vi "merge configuration with system.vi"(8 "error in":errorcluster, 11 "Scan Engine configuration in":refnum<class "Scan Engine configuration.lvclass">) -> (0 "error out":errorcluster, 3 "Scan Engine configuration out":refnum<class "Scan Engine configuration.lvclass">)   [LabVIEW 2014, in "Scan Engine runtime.lvclass"]
uses:
  Scan Engine runtime.lvclass
  <vilib>/NI/Tag Bus Module Framework/channel/channel classification.ctl
  <vilib>/NI/Tag Bus Module Framework/channel/TBM channel.lvclass
  configuration/Line.ctl
  configuration/Scan Engine configuration.lvclass
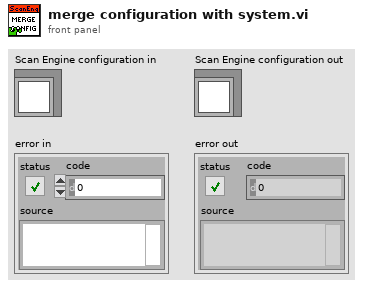
[diagram p1: front panel]
types:
  T1 = typedef "Scan Engine runtime.lvclass/system variable.ctl" = cluster{"reference":refnum<k21>, "data type":T2, "Writable":bool}
  T2 = typedef "tag bus.lvlib/tag descriptor.lvclass/Data Type.ctl" = enum16{"Double", "Single", "I64", "I32", "I16", "I8", "U64", "U32", "U16", "U8", "Boolean", "String", "Array of Double", "Array of Single", "Array of I64", "Array of I32", "Array of I16", "Array of I8", "Array of U64", "Array of U32", "Array of U16", "Array of U8", "Array of Boolean", "Array of String"}
  T3 = typedef "Scan Engine configuration.lvclass/Line.ctl" = cluster{"channel":refnum<class "TBM channel.lvclass">, "Tag":string}
  T4 = typedef "TBM channel.lvclass/channel classification.ctl" = enum16{"input data", "output data", "processing parameter", "processing result"}
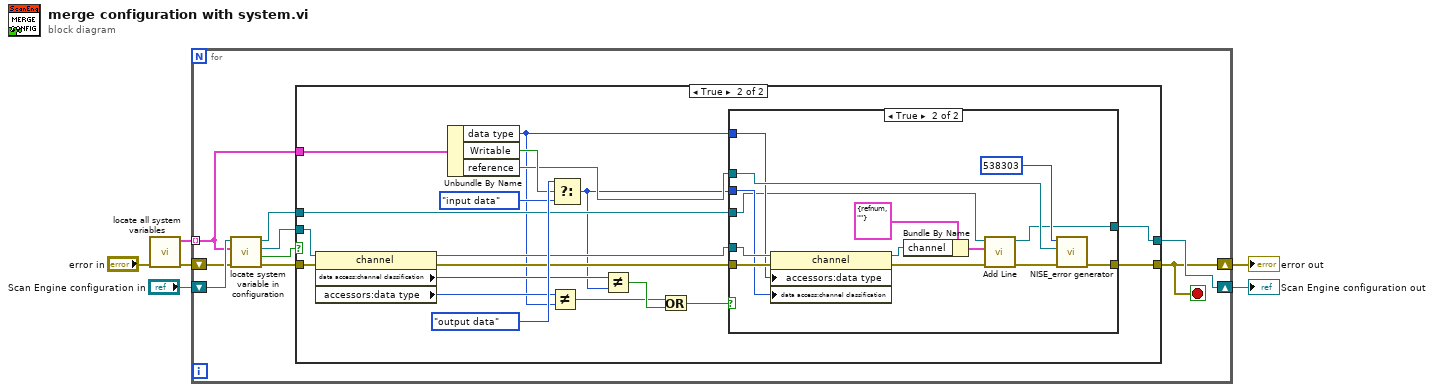
[diagram p0: block diagram]
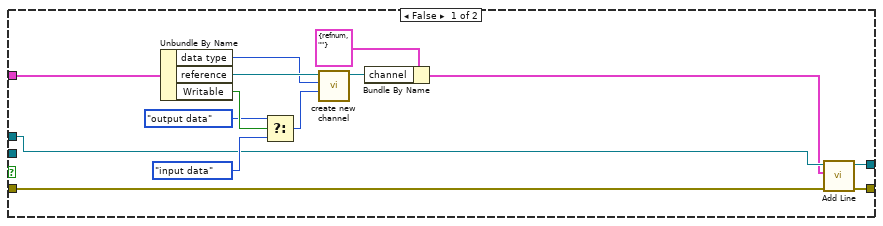
[diagram p2: hidden frame]
diagram:
  n1 = call "locate all system variables.vi"("error in"="error in") -> ("error out"=w1:errorcluster, "system variables"=w3:T1[])  [unwired: 9 in]
  n2 = for {
    shift-right: [w8] -> w5
    shift-left: "Scan Engine configuration in" -> [w15]
    shift-right: [w7] -> w4
    shift-left: w1 -> [w14]
    tunnel: w3 -> [w9] mode=indexing
    stop <- w7 stop-if-true
    n3 = call "locate system variable in configuration.vi"("error in"=w14, "raw variable data"=w9, "Scan Engine configuration in"=w15) -> ("error out"=w12:errorcluster, "found?"=w13:bool, "channel"=w10:refnum<class "TBM channel.lvclass">, "Scan Engine configuration out"=w11:refnum<class "Scan Engine configuration.lvclass">)  [unwired: 5 in]
    n4 = case shown="True" w13 {
      tunnel: w12 -> [w28 w44]
      tunnel: w11 -> [w18 w36]
      tunnel: w10 -> [_ w43]
      tunnel: w9 -> [w29 w48]
      tunnel: [w16 w34] -> w7
      tunnel: [w19 w37] -> w8
      frame False {
        n5 = Unbundle By Name(w29) -> ("data type"=w22:T2, "reference"=w23:refnum<k21>, "Writable"=w27:bool)
        n6 = Select(t=channel_classification."output data" ("channel classification"), s=w27, f=channel_classification."input data" ("channel classification")) -> (s? t:f=w24:T4)
        n7 = call <vilib>:"create new channel.vi"("channel classification"=w24, "data type"=w22, "channel name"=w23) -> ("channel"=w20:refnum<class "TBM channel.lvclass">)  [unwired: 8 in]
        n8 = Bundle By Name(cluster=T3 {"channel"=refnum, "Tag"=""} ("Line"), "channel"=w20) -> (w17:T3)
        n9 = call "Add Line.vi"("error in"=w28, "Line"=w17, "Scan Engine configuration in"=w18) -> ("error out"=w16:errorcluster, "Scan Engine configuration out"=w19:refnum<class "Scan Engine configuration.lvclass">)  [unwired: 7 in]
      }
      frame True {
        n10 = property class="channel"(reference=w43, error in=w44) -> (reference out=w32:refnum<class "TBM channel.lvclass">, error out=w35:errorcluster, "data access:channel classification"=w41:T4, "accessors:data type"=w42:T2)
        n11 = Unbundle By Name(w48) -> ("data type"=w30:T2, "Writable"=w45:bool, "reference"=w33:refnum<k21>)
        n12 = Not Equal?(x=w42, y=w30) -> (x != y?=w39:bool)
        n13 = Select(t=channel_classification."output data" ("channel classification"), s=w45, f=channel_classification."input data" ("channel classification")) -> (s? t:f=w31:T4)
        n14 = Not Equal?(x=w41, y=w31) -> (x != y?=w40:bool)
        n15 = Or(x=w39, y=w40) -> (x .or. y?=w38:bool)
        n16 = case shown="True" w38 {
          tunnel: [w50 w56] -> w37
          tunnel: w36 -> [w50 w57]
          tunnel: w35 -> [w49 w60]
          tunnel: [w49 w63] -> w34
          tunnel: w33 -> [_ w62]
          tunnel: w32 -> [_ w61]
          tunnel: w31 -> [_ w58]
          tunnel: w30 -> [_ w59]
          frame False {
          }
          frame True {
            n17 = property class="channel"(reference=w61, error in=w60, "accessors:data type"=w59, "data access:channel classification"=w58) -> (reference out=w54:refnum<class "TBM channel.lvclass">, error out=w52:errorcluster)
            n18 = Bundle By Name(cluster=T3 {"channel"=refnum, "Tag"=""} ("Line"), "channel"=w54) -> (w53:T3)
            n19 = call "Add Line.vi"("error in"=w52, "Line"=w53, "Scan Engine configuration in"=w57) -> ("error out"=w51:errorcluster, "Scan Engine configuration out"=w56:refnum<class "Scan Engine configuration.lvclass">)  [unwired: 7 in]
            n20 = call <vilib>:"NISE_error generator.vi"("error in"=w51, "append error message"=w62, "error code (0)"=538303) -> ("error out"=w63:errorcluster)  [unwired: 6 in]
          }
        }
      }
    }
  }
  "Scan Engine configuration out" <- w5
  "error out" <- w4
